vi "Remove Messages.vi"(11 "nData in":refnum<class "SOAP Data.lvclass">) -> (3 "nData out":refnum<class "SOAP Data.lvclass">)   [LabVIEW 2017, in "Controller.lvlib" / "SOAP Data.lvclass"]
uses:
  SOAP Data.lvclass
panel:
  in  "number":i32
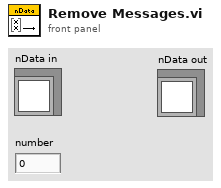
[diagram p1: front panel]
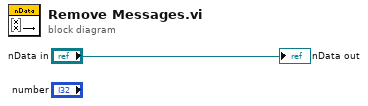
[diagram p0: block diagram]
diagram:
  "nData out" <- "nData in"
